vi "Read SSI Encoder.vi"(11 "EncoderReader in":refnum<class "EncoderReader.lvclass">) -> (2 "SSI Encoder":i32, 3 "EncoderReader out":refnum<class "EncoderReader.lvclass">)   [LabVIEW 2013, in "EncoderReader.lvlib" / "EncoderReader.lvclass"]
uses:
  <userlib>/Common/Devices/EncoderReader/EncoderReader/EncoderReader.lvclass
  <userlib>/Common/Devices/EncoderReader/EncoderReader/EncoderReader.lvclass/EncoderReader.ctl
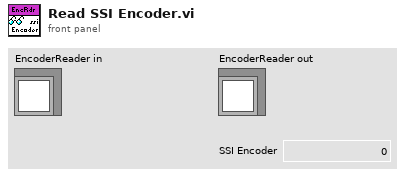
[diagram p1: front panel]
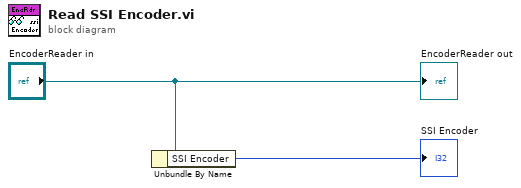
[diagram p0: block diagram]
diagram:
  n1 = Unbundle By Name("EncoderReader in") -> ("SSI Encoder"=→"SSI Encoder":i32)
  "EncoderReader out" <- "EncoderReader in"
